vi "Polynomkoeffizienten PMA.vi"() -> ()   [LabVIEW 2020, in "ABB-EL3000.lvlib" / "PMA.lvlib" / "Kalibrieren.lvlib"]
uses:
  Kalibrieren.lvlib
  Allgemeine VI/FGV Uras26 Aktion.ctl
  Allgemeine VI/Allgemeine VI.lvlib
  Allgemein/allgemeine Sub-VIs.lvlib
panel:
  in  "Abbrechen":bool
  in  "Speichern":bool
  in  "Aktiv":bool
  in  "Polynomkoeffizienten":sgl[](array[numeric])
  # "Polynomkoeffizienten PMA"
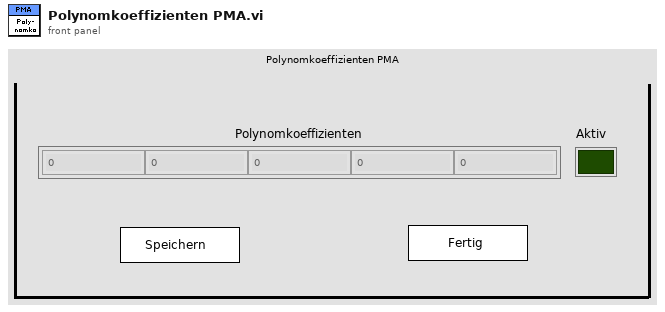
[diagram p1: front panel]
types:
  T1 = typedef "ABB-EL3000.lvlib/Allgemeine VI.lvlib/FGV Uras26 Aktion.ctl" = enum16{"lesen", "CAL-Daten laden", "Messen", "Kalibrieren vorbereiten", "Kalibrieren", "CAL-Daten speichern", "Toleranz schreiben", "CAL-Daten kopieren"}
  T2 = typedef "ABB-EL3000.lvlib/Allgemeine VI.lvlib/FGV Uras26 Aktion.ctl" = enum16{"lesen", "CAL-Daten laden", "Messen", "Kalibrieren vorbereiten", "Kalibrieren", "CAL-Daten speichern", "Toleranz schreiben", "CAL-Daten kopieren", "Polynom", "LIN aktiv", "Polynom Daten speichern", "Rohwert vor Lin", "Rohwert nach Lin"}
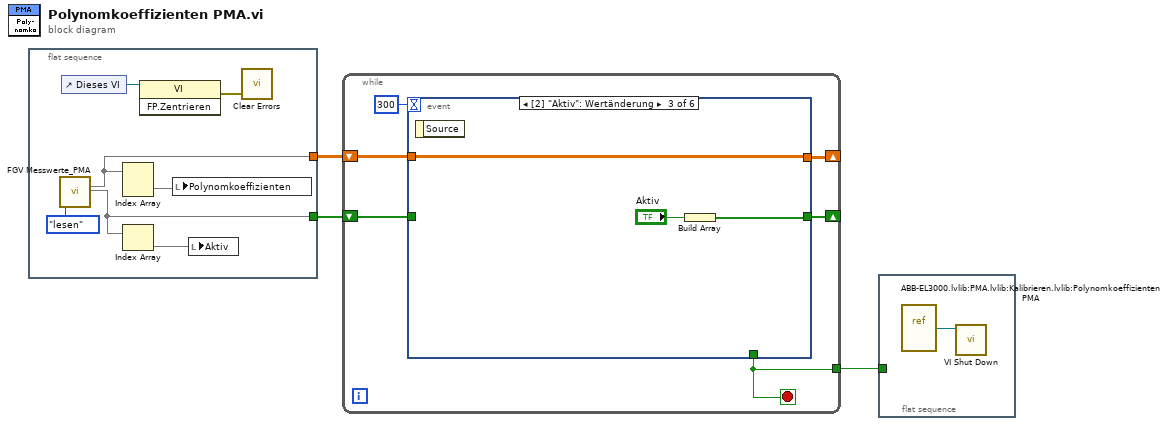
[diagram p0: block diagram]
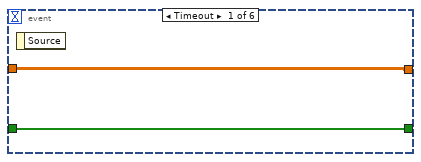
[diagram p2: hidden frame]
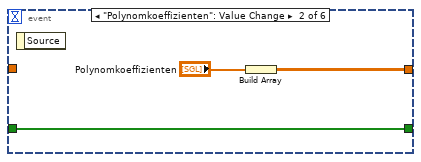
[diagram p3: hidden frame]
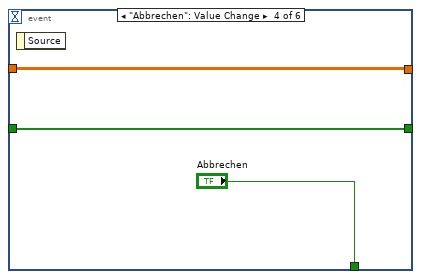
[diagram p4: hidden frame]
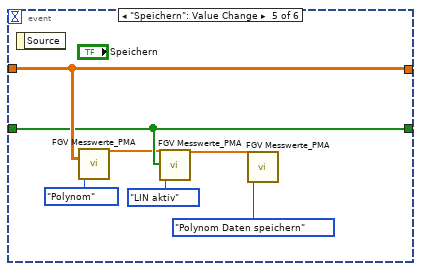
[diagram p5: hidden frame]
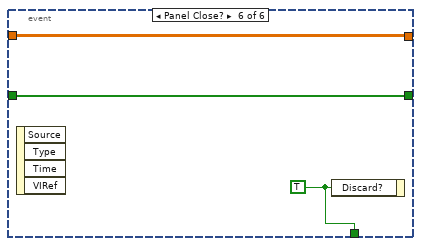
[diagram p6: hidden frame]
diagram:
  n1 = flat-sequence {
    tunnel: [w8] -> w3
    tunnel: [w7] -> w2
    frame #0 {
      n2 = call "FGV Messwerte_PMA.vi"("Aktion"=FGV_Uras26_Aktion."lesen") -> (22:w8, 23:w7)  [unwired: 17 in, 8 out]
      n3 = control-ref of="Dieses VI"() -> (w5:refnum<vi>)
      n4 = Index Array(array=w8) -> (element=w9)  [unwired: 2 in]
      n5 = Index Array(array=w7) -> (element=w6)  [unwired: 1 in]
      n6 = invoke class="VI" method="FP.Zentrieren"(reference=w5) -> (error out=w4:errorcluster)  [unwired: 2 in, 2 out]
      n7 = local write "Polynomkoeffizienten"(w9) -> ()
      n8 = local write "Aktiv"(w6) -> ()
      n9 = call <vilib>:"Clear Errors.vi"("error in (no error)"=w4) -> ()  [unwired: 5 in, 2 out]
    }
  }
  n10 = while {
    shift-right: [w14] -> _
    shift-left: w3 -> [w15]
    shift-right: [w12] -> _
    shift-left: w2 -> [w13]
    tunnel: [w11] -> w1
    stop <- w11 stop-if-true
    n11 = event shown="[2] \"Aktiv\": Wertänderung" {
      selector: _ -> [_ _ _ _ _ _]
      dyn-events: _ -> [_ _ _ _ _ _]
      timeout: 300 -> [_ _ _ _ _ _]
      tunnel: w15 -> [w18 _ w23 w27 w33 w35]
      tunnel: [w18 w19 w23 w27 w33 w35] -> w14
      tunnel: w13 -> [w17 w20 _ w26 w31 w36]
      tunnel: [w17 w20 w22 w26 w31 w36] -> w12
      tunnel: [_ _ _ "Abbrechen" _ w37] -> w11
      event Timeout {
        n12 = event-data() -> ()  [unwired: 1 in, 1 out]
      }
      event "Polynomkoeffizienten": Value Change {
        n13 = event-data() -> ()  [unwired: 1 in, 1 out]
        n14 = Build Array("Polynomkoeffizienten") -> (w19:sgl[][])
      }
      event "Aktiv": Value Change {
        n15 = event-data() -> ()  [unwired: 1 in, 1 out]
        n16 = Build Array("Aktiv") -> (w22:bool[])
      }
      event "Abbrechen": Value Change {
        n17 = event-data() -> ()  [unwired: 1 in, 1 out]
      }
      event "Speichern": Value Change {
        n18 = event-data() -> ()  [unwired: 1 in, 1 out]
        n19 = call "FGV Messwerte_PMA.vi"(2:w33, "Aktion"=FGV_Uras26_Aktion."Polynom") -> ("GasValue"=w30:sgl[])  [unwired: 18 in, 7 out]
        n20 = call "FGV Messwerte_PMA.vi"("GasValue"=w30, 3:w31, "Aktion"=FGV_Uras26_Aktion."LIN aktiv") -> ("GasValue"=w28:sgl[])  [unwired: 17 in, 7 out]
        n21 = call "FGV Messwerte_PMA.vi"("GasValue"=w28, "Aktion"=FGV_Uras26_Aktion."Polynom Daten speichern") -> ()  [unwired: 18 in, 8 out]
      }
      event Panel Close? {
        w37 = TRUE ("Verwerfen?")
        n22 = event-data() -> ()  [unwired: 1 in, 4 out]
        n23 = event-data("Discard?"=w37) -> ()  [unwired: 1 in, 1 out]
      }
    }
  }
  n24 = flat-sequence {
    tunnel: w1 -> [_]
    frame #0 {
      n25 = vi-ref "ABB-EL3000.lvlib:PMA.lvlib:Kalibrieren.lvlib:Polynomkoeffizienten PMA.vi"() -> (w38:refnum<vi>)
      n26 = call "VI Shut Down.vi"("VI Referenz"=w38) -> ()  [unwired: 11 in]
    }
  }
